vi "move.vi"(3 "error in (no error)":errorcluster, 4 "P01":dbl[](array[numeric]), 5 "P0":dbl[](array[numeric]), 6 "UART PORT in":refnum<visa-resource-name>) -> (0 "error out":errorcluster, 1 "P1":dbl[](array[numeric]), 2 "UART PORT out":refnum<visa-resource-name>)   [LabVIEW 2016]
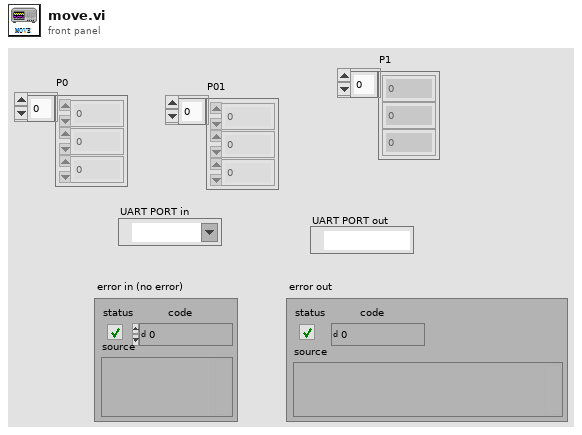
[diagram p1: front panel]
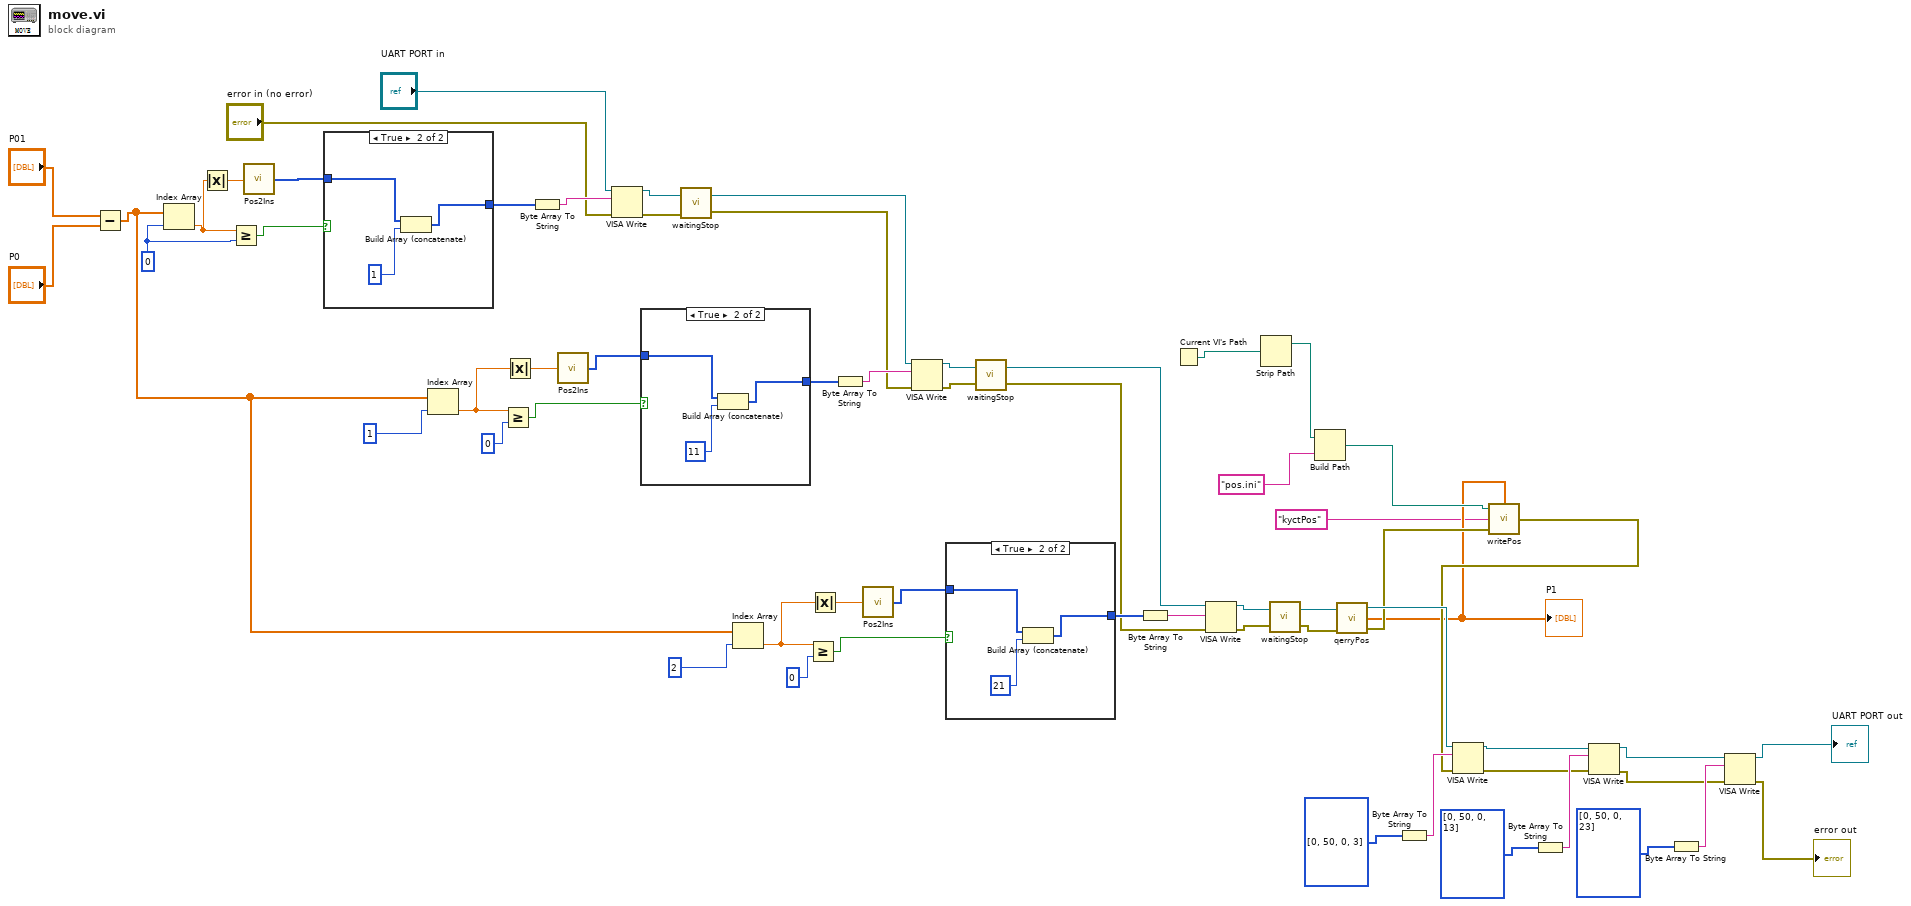
[diagram p0: block diagram]
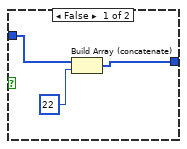
[diagram p2: hidden frame]
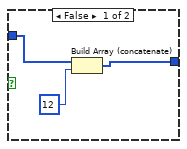
[diagram p3: hidden frame]
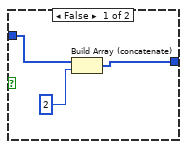
[diagram p4: hidden frame]
diagram:
  w59 = 0
  n1 = Subtract(x="P01", y="P0") -> (x-y=w29:dbl[])
  n2 = Index Array(array=w29, index=w59) -> (element=w57:dbl)
  n3 = Absolute Value(x=w57) -> (abs(x)=w56:dbl)
  n4 = Greater Or Equal?(x=w57, y=w59) -> (x >= y?=w58:bool)
  n5 = call "Pos2Ins.vi"("Pos"=w56) -> ("Ins"=w55:i32[])
  n6 = case shown="True" w58 {
    tunnel: w55 -> [w64 w67]
    tunnel: [w62 w65] -> w54
    frame False {
      n7 = Build Array (concatenate)(w64, 2) -> (w62:i32[])
    }
    frame True {
      n8 = Build Array (concatenate)(w67, 1) -> (w65:i32[])
    }
  }
  n9 = Index Array(array=w29, index=1) -> (element=w46:dbl)
  n10 = Greater Or Equal?(x=w46, y=0) -> (x >= y?=w43:bool)
  n11 = Absolute Value(x=w46) -> (abs(x)=w45:dbl)
  n12 = Byte Array To String(unsigned byte array=w54) -> (string=w53:string)
  n13 = call "Pos2Ins.vi"("Pos"=w45) -> ("Ins"=w44:i32[])
  n14 = VISA Write(VISA resource name="UART PORT in", write buffer=w53, error in (no error)="error in (no error)") -> (VISA resource name out=w50:refnum<visa-resource-name>, error out=w49:errorcluster)  [unwired: 1 out]
  n15 = case shown="True" w43 {
    tunnel: w44 -> [w70 w73]
    tunnel: [w68 w71] -> w42
    frame False {
      n16 = Build Array (concatenate)(w70, 12) -> (w68:i32[])
    }
    frame True {
      n17 = Build Array (concatenate)(w73, 11) -> (w71:i32[])
    }
  }
  n18 = call "waitingStop.vi"("error in (no error)"=w49, "UART in"=w50) -> ("error out"=w40:errorcluster, "UART out"=w39:refnum<visa-resource-name>)
  n19 = Index Array(array=w29, index=2) -> (element=w34:dbl)
  n20 = Greater Or Equal?(x=w34, y=0) -> (x >= y?=w31:bool)
  n21 = Absolute Value(x=w34) -> (abs(x)=w33:dbl)
  n22 = Byte Array To String(unsigned byte array=w42) -> (string=w41:string)
  n23 = call "Pos2Ins.vi"("Pos"=w33) -> ("Ins"=w32:i32[])
  n24 = VISA Write(VISA resource name=w39, write buffer=w41, error in (no error)=w40) -> (VISA resource name out=w38:refnum<visa-resource-name>, error out=w37:errorcluster)  [unwired: 1 out]
  n25 = case shown="True" w31 {
    tunnel: w32 -> [w76 w79]
    tunnel: [w74 w77] -> w30
    frame False {
      n26 = Build Array (concatenate)(w76, 22) -> (w74:i32[])
    }
    frame True {
      n27 = Build Array (concatenate)(w79, 21) -> (w77:i32[])
    }
  }
  n28 = call "waitingStop.vi"("error in (no error)"=w37, "UART in"=w38) -> ("error out"=w24:errorcluster, "UART out"=w25:refnum<visa-resource-name>)
  n29 = Byte Array To String(unsigned byte array=w30) -> (string=w26:string)
  n30 = Current VI's Path() -> (path=w2:path)
  n31 = VISA Write(VISA resource name=w25, write buffer=w26, error in (no error)=w24) -> (VISA resource name out=w28:refnum<visa-resource-name>, error out=w27:errorcluster)  [unwired: 1 out]
  n32 = Strip Path(path=w2) -> (stripped path=w1:path)  [unwired: 1 out]
  n33 = call "waitingStop.vi"("error in (no error)"=w27, "UART in"=w28) -> ("error out"=w22:errorcluster, "UART out"=w23:refnum<visa-resource-name>)
  n34 = Build Path(base path=w1, name or relative path="pos.ini") -> (appended path=w7:path)
  n35 = call "qerryPos.vi"("error in (no error)"=w22, "UART in"=w23) -> ("error out"=w6:errorcluster, "Array"=w4:dbl[], "UART out"=w9:refnum<visa-resource-name>)  [unwired: 2 in]
  "P1" <- w4
  n36 = Byte Array To String(unsigned byte array=i32[] [0, 50, 0, 3]) -> (string=w20:string)
  n37 = call "writePos.vi"("Pos"=w4, "error in (no error)"=w6, "name"="kyctPos", "ini Path in"=w7) -> ("error out"=w5:errorcluster)
  n38 = VISA Write(VISA resource name=w9, write buffer=w20, error in (no error)=w5) -> (VISA resource name out=w17:refnum<visa-resource-name>, error out=w16:errorcluster)  [unwired: 1 out]
  n39 = Byte Array To String(unsigned byte array=i32[] [0, 50, 0, 13]) -> (string=w18:string)
  n40 = VISA Write(VISA resource name=w17, write buffer=w18, error in (no error)=w16) -> (VISA resource name out=w12:refnum<visa-resource-name>, error out=w13:errorcluster)  [unwired: 1 out]
  n41 = Byte Array To String(unsigned byte array=i32[] [0, 50, 0, 23]) -> (string=w14:string)
  n42 = VISA Write(VISA resource name=w12, write buffer=w14, error in (no error)=w13) -> (VISA resource name out=→"UART PORT out":refnum<visa-resource-name>, error out=→"error out":errorcluster)  [unwired: 1 out]
